vi "niRFSysCalReader Cal Table Variant Name.vi"() -> (3 "Calibration Table Name":string)   [LabVIEW 2016, in "niRFSysCalReader.lvlib"]
uses:
  niRFSysCalReader.lvlib
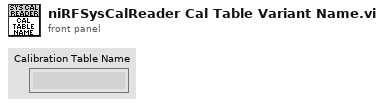
[diagram p1: front panel]
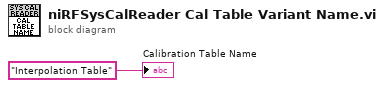
[diagram p0: block diagram]
diagram:
  "Calibration Table Name" <- "Interpolation Table" ("name")
